vi "Global LED.vi"() -> ()   [LabVIEW 2015]
panel:
  out "H_BUSY":bool[](array[boolean])
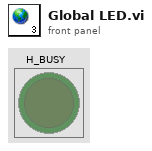
[diagram p1: front panel]
diagram:
